vi "Annotations Tip Strip.vi"(2 "Annotations Tip Strip loop ID":T1, 11 "error in (no error)":errorcluster) -> ()   [LabVIEW 2011]
uses:
  Application Structure/Loop ID.ctl
  Annotation/Actin Annotatino Holder.ctl
  emi Lib/System 01/0 - General/App/Loop control 2/Private/_emi_ SMLoop start condition.vi
  emi Lib/System 01/0 - General/App/Loop control 2/Private/_emi_ SMLoop Error Check.vi
  emi Lib/Basic/0 - General/Error/emi_Is Error.vi
  emi Lib/System 01/0 - General/App/Loop control 2/Private/_emi_SMLoop Register new.vi
  emi Lib/System 01/0 - General/S&E reporting/emi_Send S&E Error message.vi
  emi Lib/Basic/0 - General/Error/emi_ Is Error state.vi
  emi Lib/System 01/0 - General/emi_Read System ID.vi
  emi Lib/System 01/0 - General/App/Loop control/Private/_emi_GFV Loop Linking.vi
  emi Lib/System 01/0 - General/App/Loop control/Private/_emi_GFV Loop Enable.vi
  emi Lib/System 01/0 - General/App/Loop control 2/Private/_emi_ SMLoop Restart.vi
  emi Lib/System 01/0 - General/App/Private/_emi_GFV App Close.vi
  emi Lib/System 01/0 - General/App/Loop control 2/Private/_emi_ SMLoop Restart Counter.vi
  emi Lib/System 01/0 - General/App/Loop control/Private/_emi_GFV Loop Running.vi
  emi Lib/System 01/0 - General/Private/_emi_GFV System ID.vi
  emi Lib/System 01/0 - General/S&E reporting/Private/_emi_S&E Q Generator.vi
  <vilib>/Utility/error.llb/Clear Errors.vi
  emi Lib/System 01/0 - General/App/Loop control/Private/_emi_GFV stop a loop so it can reset.vi
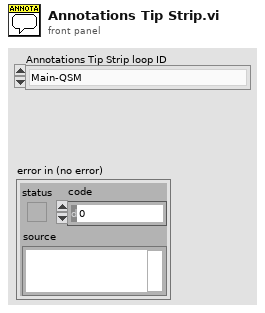
[diagram p1: front panel]
types:
  T1 = typedef "Loop ID.ctl" = enum16{"Main-QSM", "Main-Dialog", "Main-Ind Upd", "Main-Graph Upd", "Main-Debug", "Main-DebugW1", "Main-DebugW2", "Main-SE Handler", "Interface-PCP", "Interface-CANbus", "Interface-Modem", "Var Handling-Beat", "Var Handling-From PCP", "Var Handling-File storage", "Var Handling-From Simulator", "GUI-GrphW Mast", "GUI-GrphW Slav", "SIM-Tool W1", "SIM-Tool W2", "Alm-Sound", "LEIN-motor", "Tool data gatherer Qer", "Tool Data LEIN STAT2 dekoder", "Indicator Value Update", "Tool STAT2 dedicated reader", "Tool ID handler", "Detail View L1", "Detail View L2", "Main display enable view", "Sequence runner", "Voltage setpoint", "Resistance setpoint", "Stroker Wizard L1", "Stroker Wizard L2", "Alarm Handling", "Annotations Tip Strip", "Magna Interface", "Modem Status", "Var Handling - Modem Status", "Power interface detector"}
  T2 = enum16{"GET", "SET", "Get from Ini", "Put in Ini"}
  T3 = typedef "Actin Annotatino Holder.ctl" = enum16{"GET Single", "GET All", "GET Time Period", "GET Index", "Get Size", "Add Single", "Replace Single", "Delete Single", "SET All"}
  T4 = typedef "_emi_ SMLoop sates.ctl" = enum16{"Init", "Standby", "Start", "Normal Operation", "Stop", "Error Handling", "End", "Post"}
  T5 = cluster{"Minimum display time":i32, "Time set":timestamp}
  T6 = typedef "Annotations Tip Strip FGV_data cluster.ctl" = cluster{"Enabled":bool, "Point32":T7}
  T7 = typedef "LVPoint32TypeDef.ctl" = cluster{"Horizontal":i32, "Vertical":i32}
  T8 = typedef "Annotations Tip Strip FGV_cluster.ctl" = cluster{"Annotation Chart Ref":refnum<vi>, "Tip Strip Ref":refnum<vi>}
  T9 = typedef "Annotation Message.ctl" = cluster{"Annotation":string, "User":string, "time":timestamp}
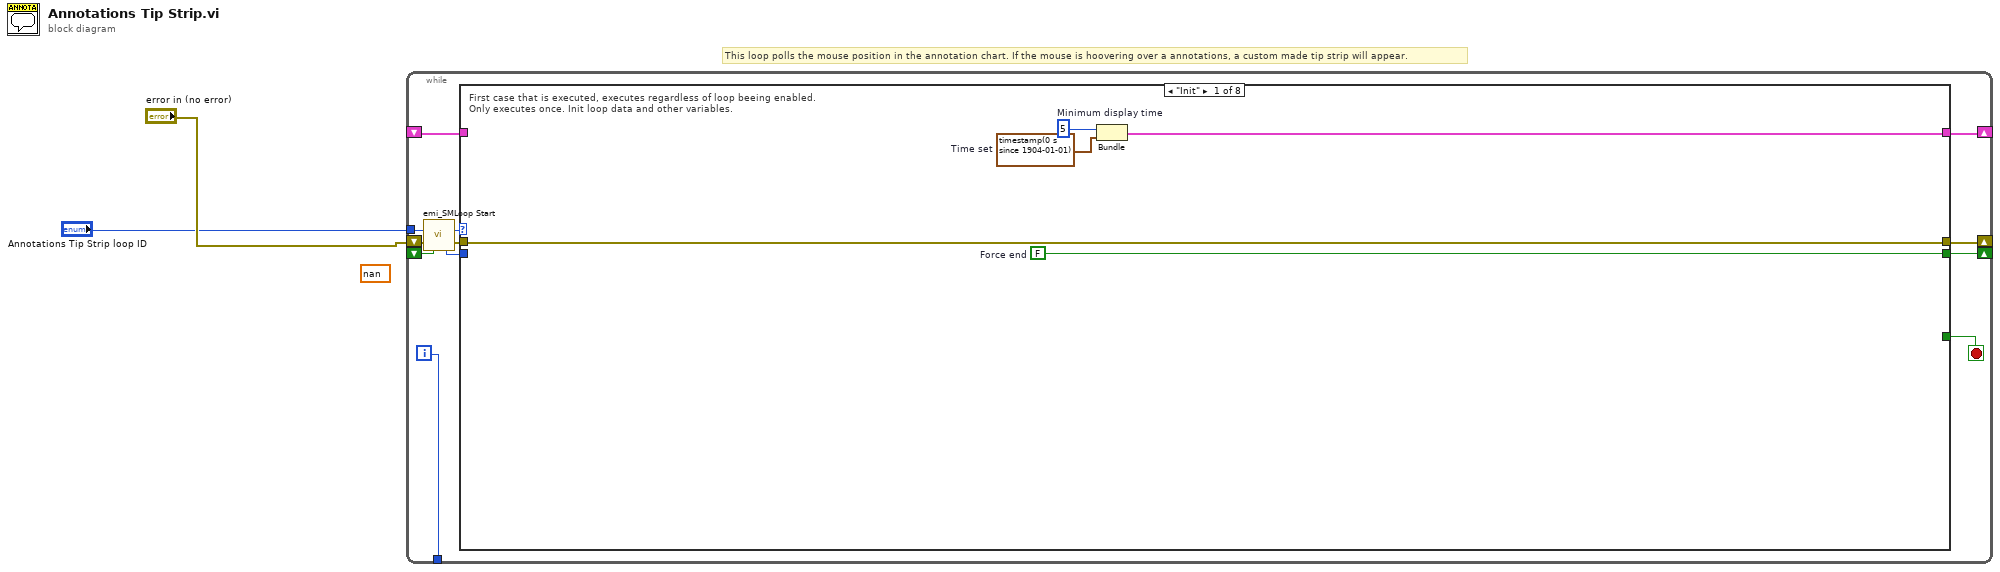
[diagram p0: block diagram]
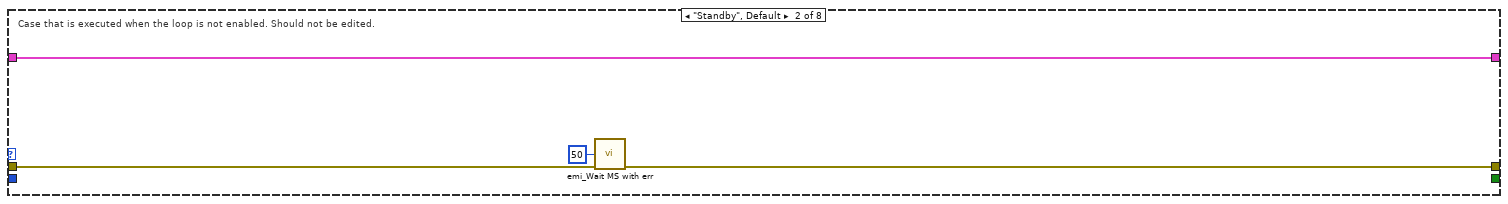
[diagram p2: hidden frame]
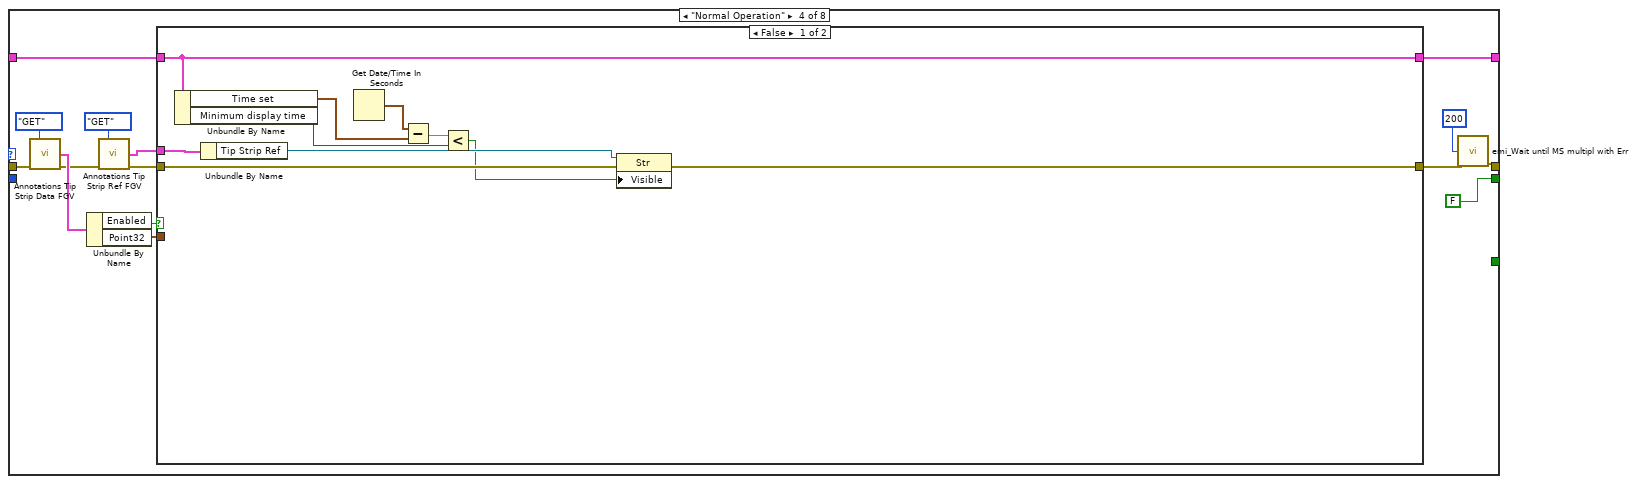
[diagram p4: hidden frame]
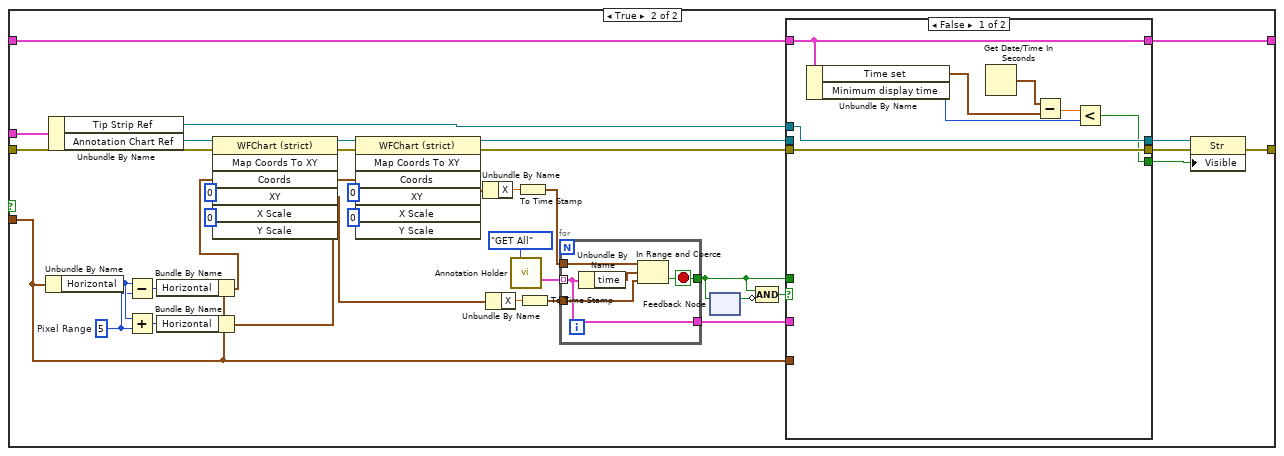
[diagram p5: hidden frame]
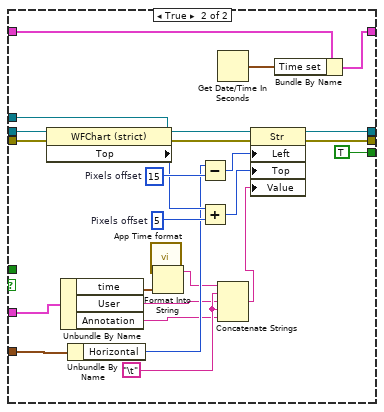
[diagram p6: hidden frame]
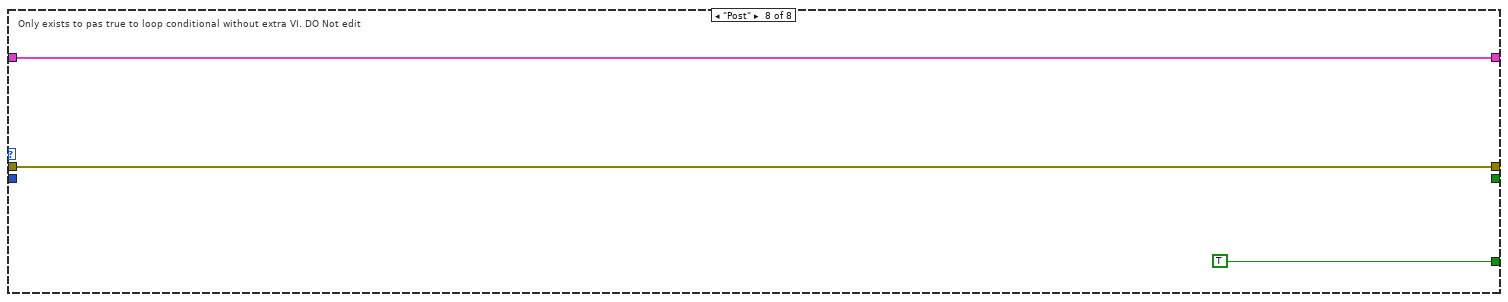
[diagram p10: hidden frame]
diagram:
  (unwired) nan
  # "This loop polls the mouse position in the annotation chart. If the mouse is hoovering over a annotations, a custom made tip strip will appear."
  n1 = while {
    shift-right: [w14] -> _
    shift-left: _ -> [w10]
    shift-right: [w12] -> _
    shift-left: "error in (no error)" -> [w8]
    tunnel: [w11] -> _
    shift-right: [w9] -> _
    shift-left: _ -> [w4]
    tunnel: "Annotations Tip Strip loop ID" -> [w5]
    i -> [w11]
    stop <- w13 stop-if-true
    n2 = call "emi_SMLoop Start.vi"("Loop ID"=w5, "error in (no error)"=w8, "Force Stop(F)"=w4) -> ("Loop command"=w6:T4, "error out"=w7:errorcluster, "Loop ID out"=w3:i32)  [unwired: 10 in]
    n3 = case shown="\"Init\"" w6 {
      tunnel: [w18 w20 w24 w26 w126 w129 w130 w133] -> w14
      tunnel: [_ _ _ _ _ _ _ TRUE] -> w13
      tunnel: w7 -> [w19 w22 w25 w35 w127 w128 w131 w134]
      tunnel: [w19 w21 w25 w39 w127 w128 w131 w134] -> w12
      tunnel: w10 -> [_ w20 w24 w27 w126 w129 w130 w133]
      tunnel: [w17 _ _ FALSE ("Force End") _ _ _ _] -> w9
      tunnel: w3 -> [_ _ _ _ _ _ _ _]
      frame "Init" {
        w15 = 5  # Minimum display time
        w16 = timestamp(0 s since 1904-01-01)  # Time set
        w17 = FALSE  # Force end
        # "First case that is executed, executes regardless of loop beeing enabled.\nOnly executes once. Init loop data and other variables."
        n4 = Bundle("Minimum display time"=w15, "Time set"=w16) -> (w18:T5)  [unwired: 1 in]
      }
      frame "Standby", Default {
        # "Case that is executed when the loop is not enabled. Should not be edited."
        n5 = call "emi_Wait MS with err.vi"("milliseconds to wait(0)"=u32 50, "error in (no error)"=w22) -> ("error out"=w21:errorcluster)  [unwired: 13 in]
      }
      frame "Start" {
        # "Start or restart the loop. Should perform any init code. \nOpen channel and so on. Will perform each time the system is restarted."
      }
      frame "Normal Operation" {
        n6 = call "Annotations Tip Strip Data FGV.vi"("Action(GET)"=T2."GET", "error in (no error)"=w35) -> ("Annotations Tip Strip Data in"=w34:T6, "error out"=w30:errorcluster)  [unwired: 12 in]
        n7 = Unbundle By Name(w34) -> ("Enabled"=w32:bool, "Point32"=w33:T7)
        n8 = call "Annotations Tip Strip Ref FGV.vi"("Action(GET)"=T2."GET", "error in (no error)"=w30) -> ("References Out"=w28:T8, "error out"=w29:errorcluster)  [unwired: 12 in]
        n9 = case shown="False" w32 {
          tunnel: [w47 w53] -> w37
          tunnel: w29 -> [w50 w58]
          tunnel: w33 -> [_ w60]
          tunnel: w28 -> [w49 w59]
          tunnel: w27 -> [w41 w56]
          tunnel: [w41 w55] -> w26
          frame False {
            n10 = Unbundle By Name(w41) -> ("Time set"=w45:timestamp, "Minimum display time"=w43:i32)
            n11 = Unbundle By Name(w49) -> ("Tip Strip Ref"=w48:refnum<vi>)
            n12 = Get Date/Time In Seconds() -> (seconds since 1Jan1904=w46:timestamp)
            n13 = Subtract(x=w46, y=w45) -> (x-y=w44:dbl)
            n14 = Less?(x=w44, y=w43) -> (x < y?=w42:bool)
            n15 = property on="Property Node" class="Str"(reference=w48, error in=w50, "Visible"=w42) -> (error out=w47:errorcluster)  [unwired: 1 out]
          }
          frame True {
            w72 = 5  # Pixel Range
            n16 = Unbundle By Name(w60) -> ("Horizontal"=w73:i32)
            n17 = Unbundle By Name(w59) -> ("Tip Strip Ref"=w61:refnum<vi>, "Annotation Chart Ref"=w62:refnum<vi>)
            n18 = Subtract(x=w73, y=w72) -> (x-y=w71:i32)
            n19 = Add(x=w73, y=w72) -> (x+y=w69:i32)
            n20 = Bundle By Name(cluster=w60, "Horizontal"=w71) -> (w70:T7)
            n21 = Bundle By Name(cluster=w60, "Horizontal"=w69) -> (w68:T7)
            n22 = invoke on="Invoke Node" class="WFChart (strict)" method="Map Coords To XY"(reference=w62, error in=w58, "Coords"=w70, "X Scale"=0, "Y Scale"=0) -> (reference out=w67:refnum<vi>, error out=w75:errorcluster, "XY"=w85:cluster{"X":dbl, "Y":dbl})  [unwired: 2 in, 4 out]
            n23 = invoke on="Invoke Node" class="WFChart (strict)" method="Map Coords To XY"(reference=w67, error in=w75, "Coords"=w68, "X Scale"=0, "Y Scale"=0) -> (reference out=w66:refnum<vi>, error out=w65:errorcluster, "XY"=w78:cluster{"X":dbl, "Y":dbl})  [unwired: 2 in, 4 out]
            n24 = Unbundle By Name(w78) -> ("X"=w79:dbl)
            n25 = Unbundle By Name(w85) -> ("X"=w84:dbl)
            n26 = call "Annotation Holder.vi"("Action"=Actin_Annotatino_Holder."GET All") -> ("Array Of annotations"=w83:T9[])  [unwired: 10 in, 4 out]
            n27 = To Time Stamp(1:w79) -> (0:w77:timestamp)
            n28 = To Time Stamp(1:w84) -> (0:w76:timestamp)
            n29 = for {
              tunnel: w83 -> [w121] mode=indexing
              tunnel: w77 -> [w125]
              tunnel: w76 -> [w124]
              tunnel: [w123] -> w64
              tunnel: [w121] -> w57
              stop <- w123 stop-if-true
              n30 = Unbundle By Name(w121) -> ("time"=w122:timestamp)
              n31 = In Range and Coerce(upper limit=w125, x=w122, lower limit=w124) -> (In Range?=w123:bool)  [unwired: 1 out]
            }
            n32 = feedback #1() -> (w63:bool)  [unwired: 1 in]
            n33 = feedback-in #1(w64) -> ()
            n34 = Compound Arithmetic op=AND(w64, invert w63) -> (w74:bool)
            n35 = case shown="False" w74 {
              tunnel: w64 -> [_ _]
              tunnel: w60 -> [_ w120]
              tunnel: w66 -> [_ w119]
              tunnel: w65 -> [w95 w118]
              tunnel: [w95 w98] -> w54
              tunnel: w61 -> [w94 w117]
              tunnel: w57 -> [_ w116]
              tunnel: w56 -> [w89 w115]
              tunnel: [w89 w114] -> w55
              tunnel: [w94 w97] -> w52
              tunnel: [w88 TRUE ("Visible")] -> w51
              frame False {
                n36 = Unbundle By Name(w89) -> ("Time set"=w92:timestamp, "Minimum display time"=w90:i32)
                n37 = Get Date/Time In Seconds() -> (seconds since 1Jan1904=w93:timestamp)
                n38 = Subtract(x=w93, y=w92) -> (x-y=w91:dbl)
                n39 = Less?(x=w91, y=w90) -> (x < y?=w88:bool)
              }
              frame True {
                w104 = "\t"
                w113 = 5  # Pixels offset
                w112 = 15  # Pixels offset
                n40 = property on="Property Node" class="WFChart (strict)"(reference=w119, error in=w118) -> (error out=w110:errorcluster, "Top"=w111:i32)  [unwired: 1 out]
                n41 = Unbundle By Name(w116) -> ("time"=w100:timestamp, "User"=w103:string, "Annotation"=w102:string)
                n42 = Unbundle By Name(w120) -> ("Horizontal"=w107:i32)
                n43 = call "App Time format.vi"() -> ("App timeformat"=w106:string)  [unwired: 15 in]
                n44 = Format Into String(format string=w106, w100) -> (resulting string=w105:string)  [unwired: 2 in, 1 out]
                n45 = Subtract(x=w107, y=w112) -> (x-y=w108:i32)
                n46 = Add(x=w111, y=w113) -> (x+y=w109:i32)
                n47 = Get Date/Time In Seconds() -> (seconds since 1Jan1904=w99:timestamp)
                n48 = Concatenate Strings(w105, w104, w103, w104, w102) -> (w101:string)
                n49 = property on="Property Node" class="Str"(reference=w117, error in=w110, "Left"=w108, "Top"=w109, "Value"=w101) -> (reference out=w97:refnum<vi>, error out=w98:errorcluster)
                n50 = Bundle By Name(cluster=w115, "Time set"=w99) -> (w114:T5)
              }
            }
            n51 = property on="Property Node" class="Str"(reference=w52, error in=w54, "Visible"=w51) -> (error out=w53:errorcluster)  [unwired: 1 out]
          }
        }
        n52 = call "emi_Wait until MS multipl with Err.vi"("millisecond multiple(0)"=u32 200, "error in (no error)"=w37) -> ("error out"=w39:errorcluster)  [unwired: 13 in]
      }
      frame "Stop" {
        # "Stop the loop. May be restarted later. Close interfaces and the like"
      }
      frame "Error Handling" {
        # "Loop automaticaly returns here after error is found. If error is cleared, \nLoop wil continue as normal(if was operative when error."
      }
      frame "End" {
        # "Only executes at application end has. Should performa any action the loop \nneeds to finnish. Executes only once."
      }
      frame "Post" {
        # "Only exists to pas true to loop conditional without extra VI. DO Not edit"
      }
    }
  }
